vi "demo-geometry.vi"() -> ()   [LabVIEW 2019]
uses:
  ROBOT_PICTURE.ctl
  <vilib>/Rock Robotics/WPI/ThirdParty/JAS_Junk/TrajLib/TypeDef/POSE2D.ctl
  <vilib>/Rock Robotics/WPI/ThirdParty/JAS_Junk/TrajLib/TypeDef/TRANSLATION2D.ctl
  <vilib>/Rock Robotics/WPI/ThirdParty/JAS_Junk/TrajLib/TypeDef/ROTATION2D.ctl
  <vilib>/Rock Robotics/WPI/ThirdParty/JAS_Junk/TrajLib/Transform_Create_PosePose.vi
  <vilib>/Rock Robotics/WPI/ThirdParty/JAS_Junk/TrajLib/Util_CalcDist.vi
  <vilib>/Rock Robotics/WPI/ThirdParty/JAS_Junk/TrajLib/Rotation_UnaryMinus.vi
  <vilib>/Rock Robotics/WPI/ThirdParty/JAS_Junk/TrajLib/Translation_RotateBy.vi
  <vilib>/Rock Robotics/WPI/ThirdParty/JAS_Junk/TrajLib/Translation_Minus.vi
  <vilib>/Rock Robotics/WPI/ThirdParty/JAS_Junk/TrajLib/Rotation_Minus.vi
  <vilib>/Rock Robotics/WPI/ThirdParty/JAS_Junk/TrajLib/Rotation_RotateBy.vi
  <vilib>/picture/pixmap.llb/Flatten Pixmap.vi
  <vilib>/picture/pictutil.llb/Create Mask.vi
  <vilib>/picture/picture.llb/Draw Flattened Pixmap.vi
  <vilib>/Rock Robotics/WPI/ThirdParty/JAS_Junk/TrajLib/Trajectory_Library.lvlib
panel:
  out "Ball Angle From Robot":T1 {"SIN" format="%13.4f"; "COS" format="%13.4f"; "VALUE" format="%13.4f"}
  out "Ball Location From Robot":T2 {"Y" format="%14.3f"; "X" format="%14.3f"}
  out "Ball Location":T2 {"Y" format="%14.3f"; "X" format="%14.3f"}
  out "Robot POSE":T3 {"ROTATION"."SIN" format="%13.4f"; "ROTATION"."COS" format="%13.4f"; "ROTATION"."VALUE" format="%13.4f"; "TRANSLATION"."Y" format="%14.3f"; "TRANSLATION"."X" format="%14.3f"}
  out "BALL":bool=TRUE
  in  "Y  INCHES - BALL":dbl=220.0
  in  "X INCHES - BALL":dbl=200.0
  in  "ORIENTATION - DEG":dbl
  in  "Y  INCHES":dbl=40.0
  in  "X INCHES":dbl=20.0
  out "2D Picture":T4
  # "ROBOT"
  # "BALL"
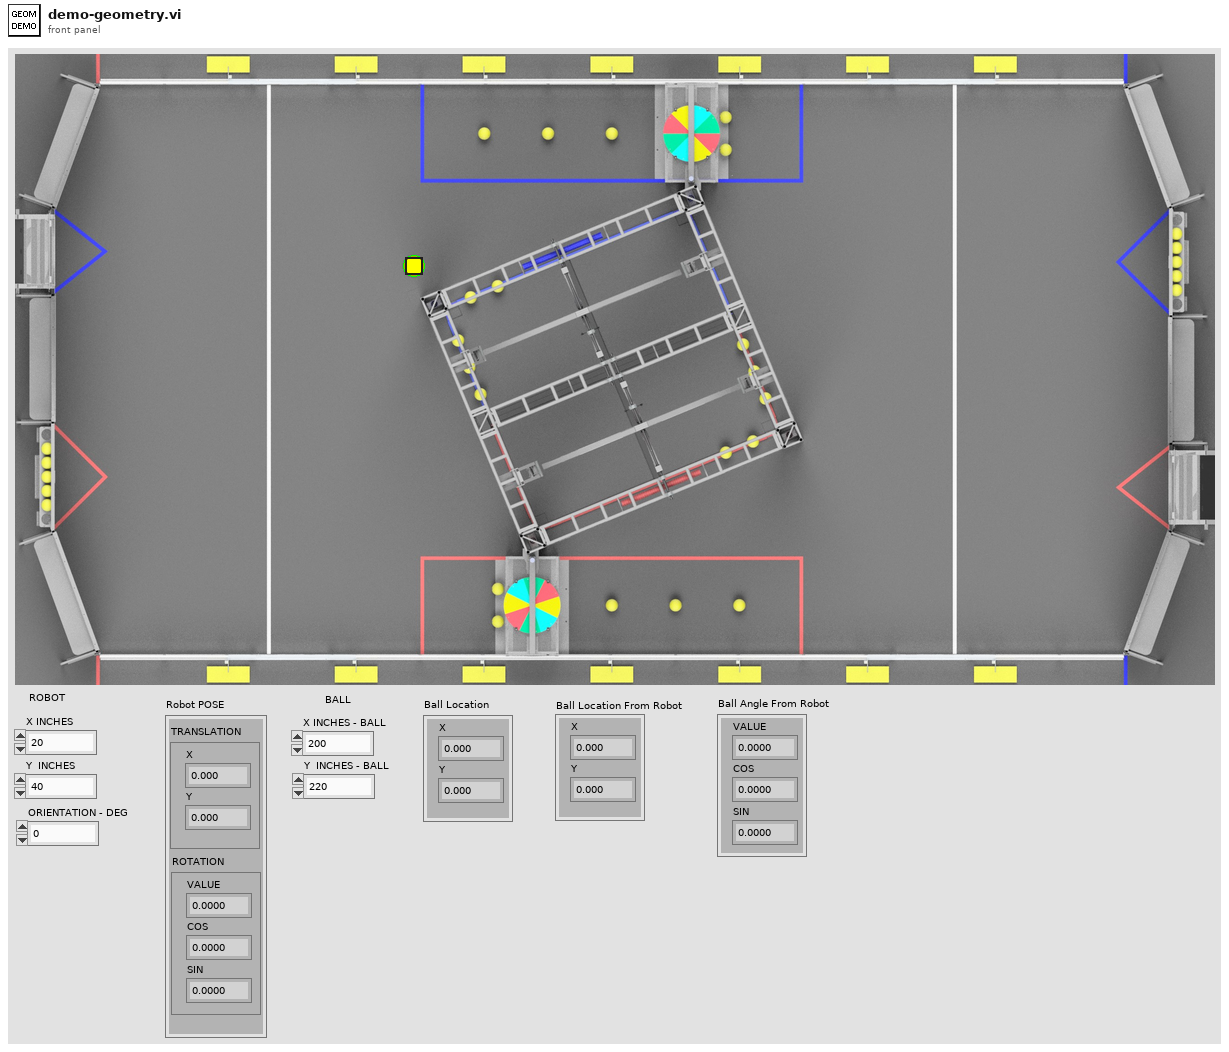
[diagram p1: front panel]
types:
  T1 = typedef "Trajectory_Library.lvlib/ROTATION2D.ctl" = cluster{"VALUE":dbl, "COS":dbl, "SIN":dbl}
  T2 = typedef "Trajectory_Library.lvlib/TRANSLATION2D.ctl" = cluster{"X":dbl, "Y":dbl}
  T3 = typedef "Trajectory_Library.lvlib/POSE2D.ctl" = cluster{"TRANSLATION":T2, "ROTATION":T1}
  T4 = typedef "ROBOT_PICTURE.ctl" = picture
  T5 = typedef "Rotated_Picture_TypeDef.ctl" = cluster{"ONE-8-bit pixmap":u8[][], "Two-Array":cdb[][], "Three-Numeric":i32, "Four-Numeric":i32, "Five-Numeric":cdb, "Six-colors":u32[], "Seven-new element/subarray":u32, "Eight-Cluster":cluster{"[0]":i32, "[1]":i32}}
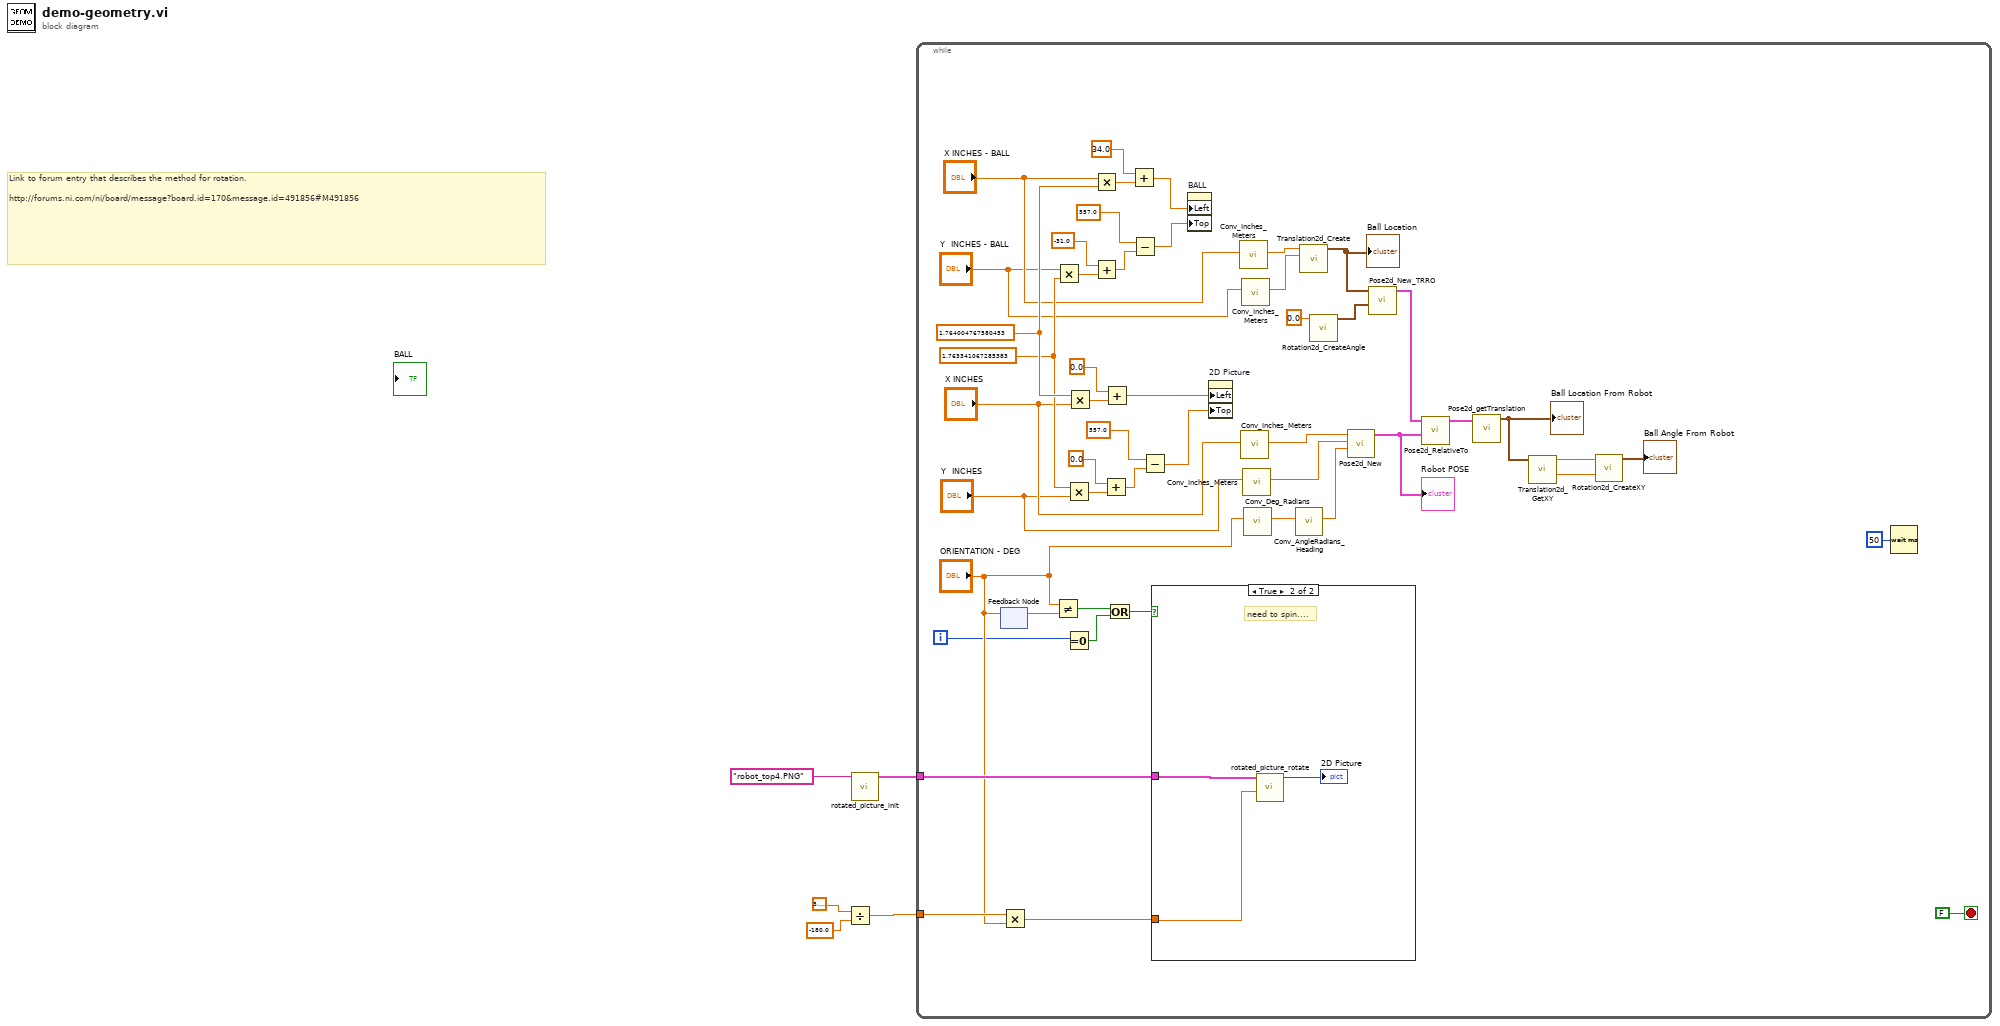
[diagram p0: block diagram]
diagram:
  # "Link to forum entry that describes the method for rotation.\n\nhttp://forums.ni.com/ni/board/message?board.id=170&message.id=491856#M491856"
  n1 = Divide(x=3.141592653589793, y=-180.0 ("value")) -> (x/y=w3:dbl)
  n2 = call "rotated_picture_init.vi"("Picture FIle Name"="robot_top4.PNG" ("name or relative path")) -> ("RotatedPictureInfo"=w1:T5)  [unwired: 10 in]
  n3 = while {
    tunnel: w3 -> [w54]
    tunnel: w1 -> [w53]
    i -> [w6]
    stop <- FALSE stop-if-true
    w31 = 1.763341067285383
    w38 = 1.764004767580453
    n4 = feedback-in #1("ORIENTATION - DEG") -> ()
    n5 = feedback #1() -> (w49:dbl)  [unwired: 1 in]
    n6 = Multiply(x=w54, y="ORIENTATION - DEG") -> (x*y=w51:dbl)
    n7 = Not Equal?(x="ORIENTATION - DEG", y=w49) -> (x != y?=w8:bool)
    n8 = Multiply(x="Y  INCHES - BALL", y=w31) -> (x*y=w36:dbl)
    n9 = Multiply(x=w31, y="Y  INCHES") -> (x*y=w46:dbl)
    n10 = Equal To 0?(x=w6) -> (x = 0?=w7:bool)
    n11 = Multiply(x=w38, y="X INCHES") -> (x*y=w48:dbl)
    n12 = Multiply(x="X INCHES - BALL", y=w38) -> (x*y=w40:dbl)
    n13 = Add(x=-31.0, y=w36) -> (x+y=w33:dbl)
    n14 = Add(x=0.0, y=w46) -> (x+y=w42:dbl)
    n15 = Add(x=0.0, y=w48) -> (x+y=w43:dbl)
    n16 = Or(x=w8, y=w7) -> (x .or. y?=w9:bool)
    n17 = Add(x=34.0, y=w40) -> (x+y=w37:dbl)
    n18 = Subtract(x=557.0, y=w33) -> (x-y=w32:dbl)
    n19 = Subtract(x=557.0, y=w42) -> (x-y=w41:dbl)
    n20 = case shown="True" w9 {
      tunnel: w53 -> [_ w56]
      tunnel: w51 -> [_ w55]
      frame False {
        # "Leave as is..."
      }
      frame True {
        # "need to spin...."
        n21 = call "rotated_picture_rotate.vi"("Angle"=w55, "RotatedPictureInfo"=w56) -> ("new picture"=→"2D Picture":picture)  [unwired: 9 in]
      }
    }
    n22 = property on="BALL" class="Bool (strict)"("Left"=w37, "Top"=w32) -> ()  [unwired: 2 in, 2 out]
    n23 = property on="2D Picture" class="Pict (strict)"("Left"=w43, "Top"=w41) -> ()  [unwired: 2 in, 2 out]
    n24 = call <vilib>:"Conv_Inches_Meters.vi"("INCH"="X INCHES - BALL") -> ("Meters"=w22:dbl)  [unwired: 10 in]
    n25 = call <vilib>:"Conv_Inches_Meters.vi"("INCH"="X INCHES") -> ("Meters"=w26:dbl)  [unwired: 10 in]
    n26 = call <vilib>:"Conv_Inches_Meters.vi"("INCH"="Y  INCHES - BALL") -> ("Meters"=w21:dbl)  [unwired: 10 in]
    n27 = call <vilib>:"Conv_Inches_Meters.vi"("INCH"="Y  INCHES") -> ("Meters"=w25:dbl)  [unwired: 10 in]
    n28 = call <vilib>:"Conv_Deg_Radians.vi"("Degress"="ORIENTATION - DEG") -> ("Radians"=w27:dbl)  [unwired: 10 in]
    n29 = call <vilib>:"Conv_AngleRadians_Heading.vi"("Radians"=w27) -> ("Heading"=w18:dbl)  [unwired: 10 in]
    n30 = call <vilib>:"Translation2d_Create.vi"("Y"=w21, "X"=w22) -> ("TRANSLATION"=w20:T2)  [unwired: 9 in]
    "Ball Location" <- w20
    n31 = call <vilib>:"Rotation2d_CreateAngle.vi"("Angle"=0.0) -> ("ROTATION"=w15:T1)  [unwired: 10 in]
    n32 = call <vilib>:"Pose2d_New.vi"("Heading"=w18, "Y"=w25, "X"=w26) -> ("out POSe"=w17:T3)  [unwired: 8 in]
    "Robot POSE" <- w17
    n33 = call <vilib>:"Pose2d_New_TRRO.vi"("ROTATION"=w15, "TRANSLATION"=w20) -> ("outPOSE"=w19:T3)  [unwired: 9 in]
    n34 = call <vilib>:"Pose2d_RelativeTo.vi"("other POSE"=w17, "in POSE"=w19) -> ("out POSE"=w14:T3)  [unwired: 9 in]
    n35 = call <vilib>:"Pose2d_getTranslation.vi"("in POSE"=w14) -> ("outTRANSLATION"=w13:T2)  [unwired: 10 in]
    "Ball Location From Robot" <- w13
    n36 = call <vilib>:"Translation2d_GetXY.vi"("In Translation"=w13) -> ("Y"=w11:dbl, "X"=w12:dbl)  [unwired: 9 in]
    n37 = call <vilib>:"Rotation2d_CreateXY.vi"("Y or sine"=w11, "X or  cosine"=w12) -> ("ROTATION"=→"Ball Angle From Robot":T1)  [unwired: 9 in]
    n38 = Wait (ms)(milliseconds to wait=u32 50) -> ()  [unwired: 1 out]
  }
